vi "Read Raw.vi"(8 "error in (no error)":errorcluster, 10 "Path":path, 11 "ImageHandler in":refnum<class "ImageHandler.lvclass">) -> (0 "error out":errorcluster, 3 "ImageHandler out":refnum<class "ImageHandler.lvclass">)   [LabVIEW 2021, in "ImageHandler.lvlib" / "ImageHandler.lvclass"]
uses:
  ImageHandler.lvclass
  ImageHandler.lvclass/ImageHandler.ctl
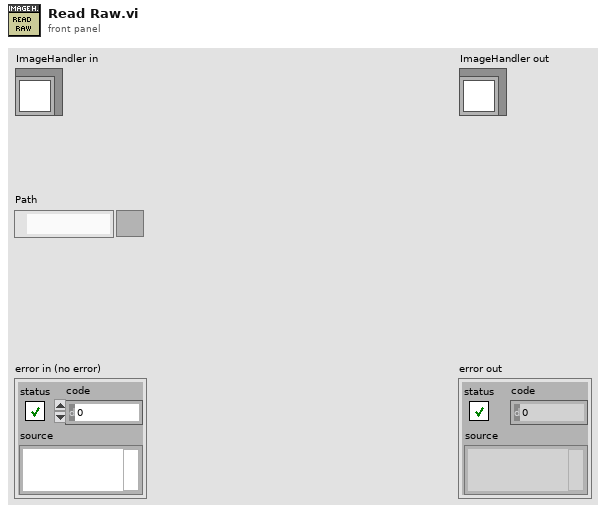
[diagram p1: front panel]
types:
  T1 = enum16{"open", "replace", "create", "open or create", "replace or create", "replace or create with confirmation"}
  T2 = typedef "IMAQ Image.ctl" = refnum<image>
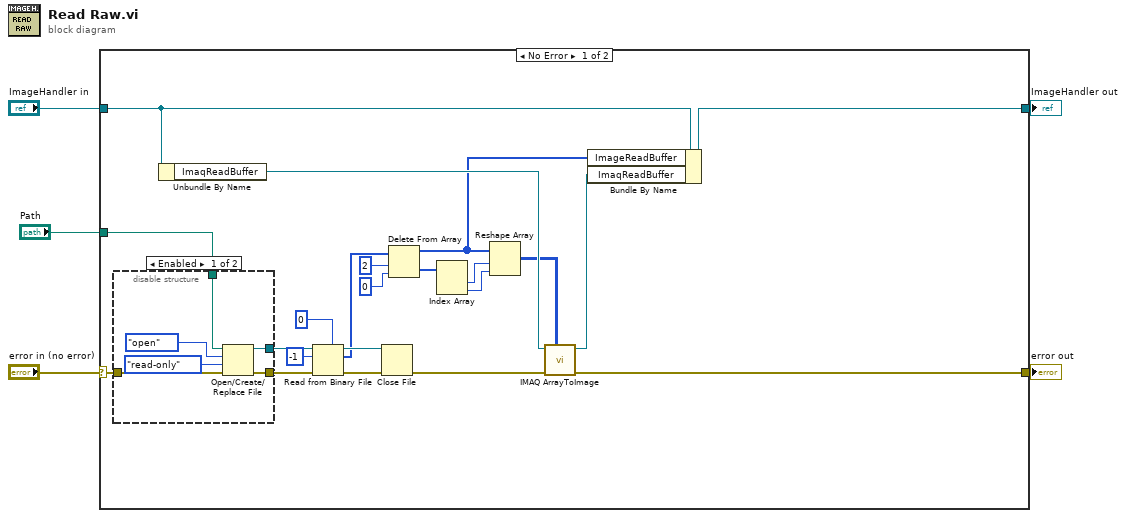
[diagram p0: block diagram]
diagram:
  n1 = case shown="No Error" "error in (no error)" {
    selector: "error in (no error)" -> [w27 w37]
    tunnel: [w9 w37] -> w4
    tunnel: [w8 w36] -> w2
    tunnel: "ImageHandler in" -> [w26 w36]
    tunnel: "Path" -> [w23 _]
    frame No Error {
      n2 = disable-structure shown="Enabled" {
        disable-tunnel: w27 -> [w33 w34]
        disable-tunnel: [w32 w34] -> w25
        disable-tunnel: w23 -> [w31 w35]
        disable-tunnel: [w30 w35] -> w22
        frame Enabled {
          n3 = Open/Create/Replace File(file path (use dialog)=w31, error in=w33, operation (0:open)=T1."open", access (0:read/write)=enum16{"read/write", "read-only", "write-only"}."read-only") -> (refnum out=w30:refnum<file>, error out=w32:errorcluster)  [unwired: 2 in, 1 out]
        }
        frame Disabled {
        }
      }
      n4 = Unbundle By Name(w26) -> ("ImaqReadBuffer"=w12:T2)
      n5 = Read from Binary File(5:u16 0, 8:w25, 10:-1 ("count (1)"), 11:w22) -> (0:w24:errorcluster, 2:w18:u16[], 3:w21:refnum<file>)  [unwired: 2 in, 1 out]
      n6 = Close File(refnum=w21, error in=w24) -> (error out=w10:errorcluster)  [unwired: 1 out]
      n7 = Delete From Array(array=w18, length=2, index=0) -> (deleted portion=w15:u16[], array with subset deleted=w6:u16[])
      n8 = Index Array(array=w15) -> (element #1=w14:u16, element #2=w13:u16)  [unwired: 2 in]
      n9 = Reshape Array(w6, w14, w13) -> (w11:u16[][])
      n10 = call "IMAQ ArrayToImage"("Image Pixels (U16)"=w11, "error in (no error)"=w10, "Image"=w12) -> ("error out"=w9:errorcluster, "Image Out"=w7:T2)  [unwired: 7 in]
      n11 = Bundle By Name(cluster=w26, "ImageReadBuffer"=w6, "ImaqReadBuffer"=w7) -> (w8:refnum<class "ImageHandler.lvclass">)
    }
    frame Error {
    }
  }
  "error out" <- w4
  "ImageHandler out" <- w2
